vi "Test Headers.vi"(8 "error in":errorcluster) -> (0 "error out":errorcluster)   [LabVIEW 2016]
uses:
  <vilib>/addons/_JKI Toolkits/Caraya/classes/Assert/Assert.lvclass
  Request/Request.lvclass
  <vilib>/addons/_JKI Toolkits/Caraya/classes/Test/Test.lvclass
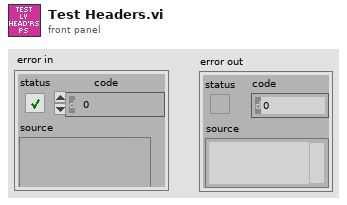
[diagram p1: front panel]
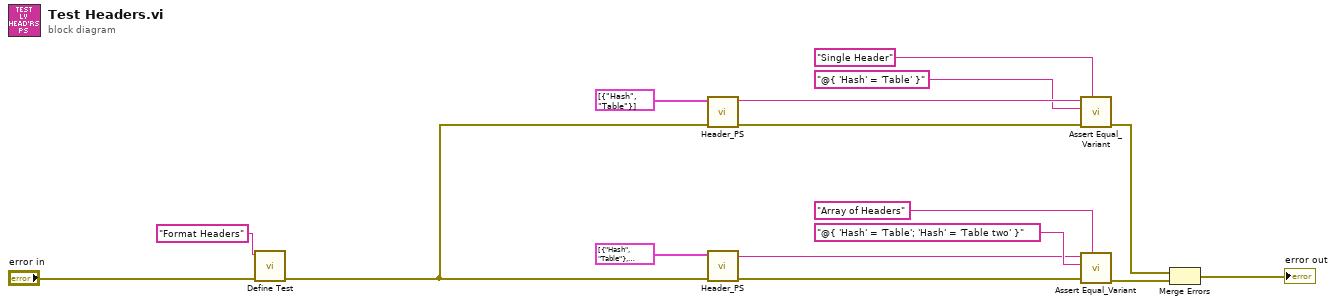
[diagram p0: block diagram]
diagram:
  n1 = call <vilib>:"Define Test.vi"("error in (no error)"="error in", "Label (VI Title)"="Format Headers") -> ("error out"=w7:errorcluster)  [unwired: 9 in]
  n2 = call "Header_PS.vi"("error in"=w7, "Headers In"=cluster{"Name":string, "Value":string}[] [{"Name"="Hash", "Value"="Table"}]) -> ("error out"=w14:errorcluster, "Headers_PS_Dict"=w16:string)  [unwired: 8 in]
  n3 = call "Header_PS.vi"("error in"=w7, "Headers In"=cluster{"Name":string, "Value":string}[] [{"Name"="Hash", "Value"="Table"}, {"Name"="Hash", "Value"="Table two"}]) -> ("error out"=w6:errorcluster, "Headers_PS_Dict"=w9:string)  [unwired: 8 in]
  n4 = call <vilib>:"Assert Equal_Variant.vi"("Label"="Single Header", "error in (no error)"=w14, "Y"="@{ 'Hash' = 'Table' }", "X"=w16) -> ("error out"=w4:errorcluster)  [unwired: 7 in]
  n5 = call <vilib>:"Assert Equal_Variant.vi"("Label"="Array of Headers", "error in (no error)"=w6, "Y"="@{ 'Hash' = 'Table'; 'Hash' = 'Table two' }", "X"=w9) -> ("error out"=w5:errorcluster)  [unwired: 7 in]
  n6 = Merge Errors(w4, w5) -> (→"error out":errorcluster)
